vi "SSL_write.vi"(8 "error in (no error)":errorcluster, 10 "Write string":u8[](array[numeric]), 11 "SSL in":refnum<class "SSL.lvclass">) -> (0 "error out":errorcluster, 2 "Bytes written":i32, 3 "SSL out":refnum<class "SSL.lvclass">)   [LabVIEW 2013, in "SSL_Lib.lvlib" / "SSL.lvclass"]
uses:
  SSL.lvclass
  SSL-Lib/SSL-Lib.lvclass/SSL-Lib.ctl
  SSL.lvclass/SSL.ctl
  SSL-Lib/Read SSL Library Path.vi
  Read Handle.vi
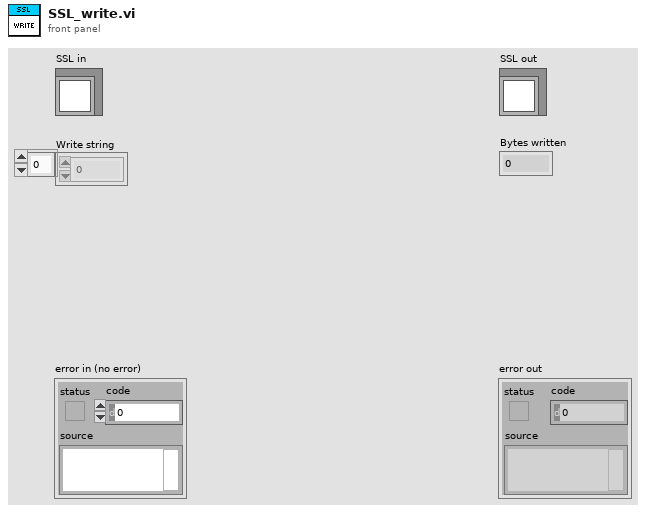
[diagram p1: front panel]
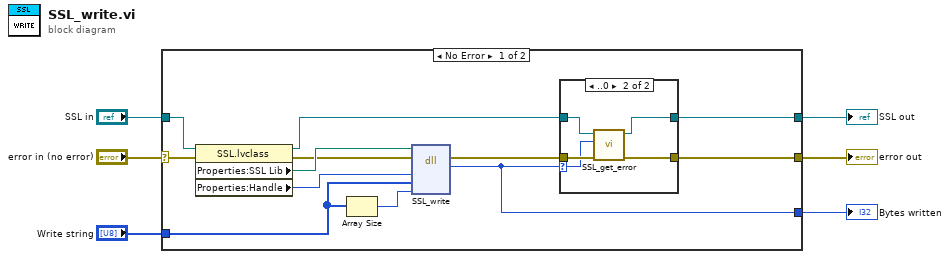
[diagram p0: block diagram]
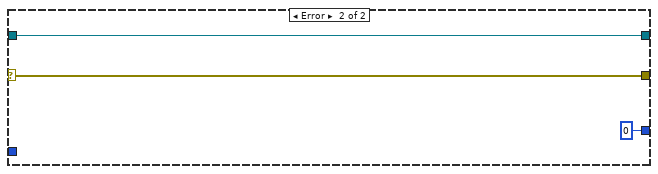
[diagram p3: hidden frame]
diagram:
  n1 = case shown="No Error" "error in (no error)" {
    selector: "error in (no error)" -> [w17 w28]
    tunnel: [w12 w28] -> w5
    tunnel: [w10 w27] -> w3
    tunnel: "SSL in" -> [w18 w27]
    tunnel: "Write string" -> [w9 _]
    tunnel: [w7 0 ("return type")] -> w1
    frame No Error {
      n2 = property class="SSL.lvclass"(reference=w18, error in=w17) -> (reference out=w11:refnum<class "SSL.lvclass">, error out=w15:errorcluster, "Properties:SSL Lib"=w16:path, "Properties:Handle"=w13:u64)
      n3 = Array Size(array=w9) -> (size(s)=w8:i32)
      n4 = dll-call lib="C:/Program Files (x86)/National Instruments/Shared/nissl/NIssleay32.dll" fn="SSL_write"(path in=w16, error in=w15, "SSL"=w13, "buf"=w9, "len"=w8) -> (error out=w14:errorcluster, "return type"=w7:i32)  [unwired: 4 in, 1 out]
      n5 = case shown="..0" w7 {
        selector: w7 -> [_ w21]
        tunnel: w14 -> [w19 w25]
        tunnel: [w19 w24] -> w12
        tunnel: w11 -> [w20 w23]
        tunnel: [w20 w22] -> w10
        frame Default {
        }
        frame ..0 {
          n6 = call "SSL_get_error.vi"("error in (no error)"=w25, "SSL return code"=w21, "SSL-Lib in"=w23) -> ("error out"=w24:errorcluster, "SSL-Lib out"=w22:refnum<class "SSL.lvclass">)  [unwired: 6 in, 1 out]
        }
      }
    }
    frame Error {
    }
  }
  "error out" <- w5
  "SSL out" <- w3
  "Bytes written" <- w1
